vi "Process Script Check.vi"(8 "error in (no error)":errorcluster, 10 "Message":T1, 11 "Tamer in":refnum<class "Tamer.lvclass">=refnum) -> (0 "error out":errorcluster, 3 "Tamer out":refnum<class "Tamer.lvclass">)   [LabVIEW 2020, in "CIRCUS_uServices.lvlib" / "Holy Trinity.lvlib" / "Tamer.lvlib" / "Tamer.lvclass"]
uses:
  Tamer.lvclass
  TALOS/TALOS_PPL.lvlibp
  Run Utilities/TypeDefs/Script Checker Result.ctl
  Run Utilities/Run Utilities.lvlib
  Run Utilities/TypeDefs/Messages/Script Checker Message.ctl
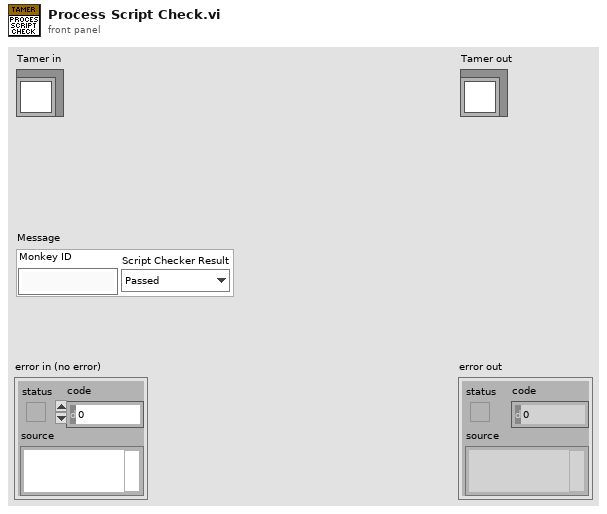
[diagram p1: front panel]
types:
  T1 = typedef "CIRCUS_uServices.lvlib/Run Utilities.lvlib/Script Checker Message.ctl" = cluster{"Monkey ID":string, "Script Checker Result":T2}
  T2 = typedef "CIRCUS_uServices.lvlib/Run Utilities.lvlib/Script Checker Result.ctl" = enum16{"Passed", "Failed", "Empty"}
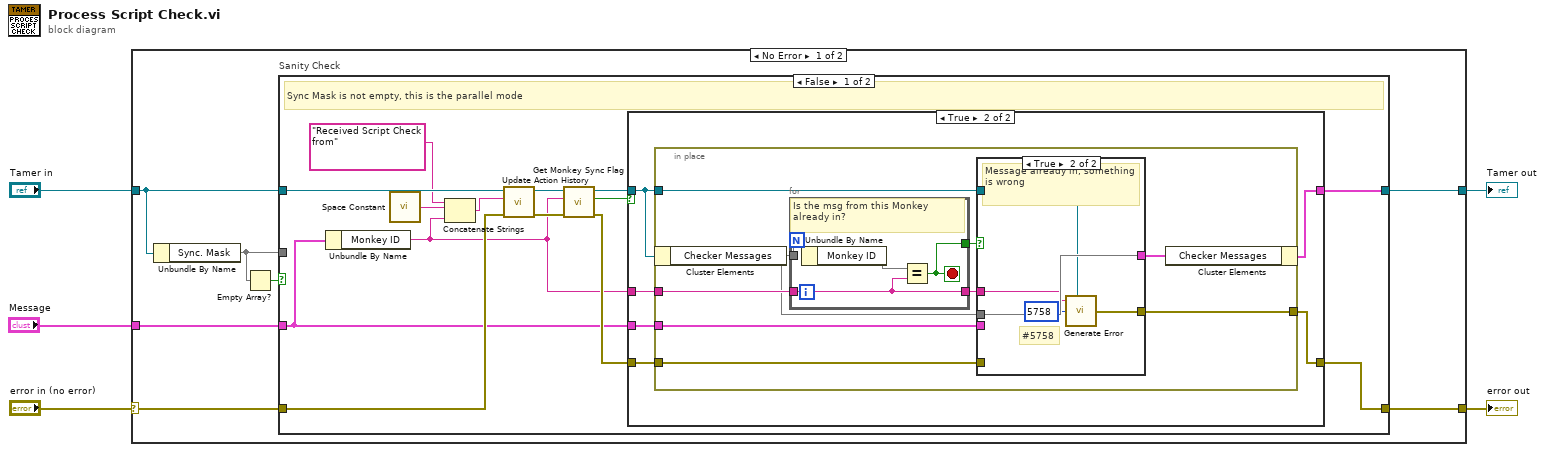
[diagram p0: block diagram]
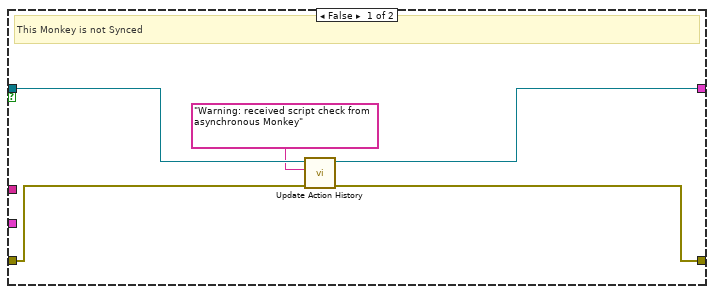
[diagram p2: hidden frame]
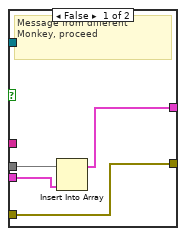
[diagram p3: hidden frame]
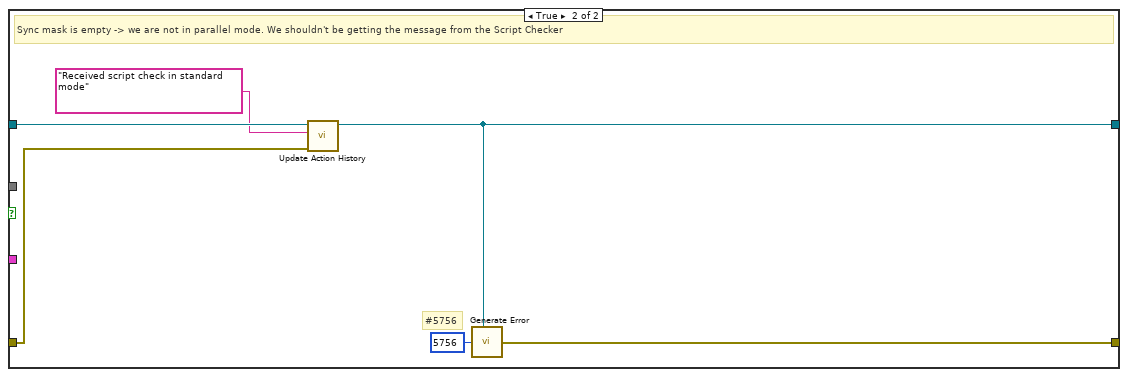
[diagram p4: hidden frame]
diagram:
  n1 = case shown="No Error" "error in (no error)" {
    selector: "error in (no error)" -> [w7 w67]
    tunnel: [w8 w67] -> w4
    tunnel: [w6 w66] -> w2
    tunnel: "Tamer in" -> [w9 w66]
    tunnel: "Message" -> [w12 _]
    frame No Error {
      n2 = Unbundle By Name(w9) -> ("Sync. Mask"=w10)
      n3 = Empty Array?(array=w10) -> (empty?=w11:bool)
      n4 = case "Sanity Check" shown="False" w11 {
        tunnel: w12 -> [w22 _]
        tunnel: w10 -> [_ _]
        tunnel: w9 -> [w18 w63]
        tunnel: [w21 w65] -> w8
        tunnel: w7 -> [w26 w60]
        tunnel: [w20 w62] -> w6
        frame False {
          # "Sync Mask is not empty, this is the parallel mode"
          n5 = Unbundle By Name(w22) -> ("Monkey ID"=w13:string)
          n6 = call <vilib>:"Space Constant.vi"() -> ("String"=w14:string)
          n7 = Concatenate Strings("Received Script Check from" ("string"), w14, w13) -> (w15:string)
          n8 = call-dynamic "Update Action History.vi"("error in (no error)"=w26, "Action"=w15, "Tamer in"=w18) -> ("error out"=w25:errorcluster, "Tamer out"=w17:refnum<class "Tamer.lvclass">)  [unwired: 7 in]
          n9 = call-dynamic "Get Monkey Sync Flag.vi"("error in (no error)"=w25, "Monkey ID"=w13, "Tamer in"=w17) -> ("error out"=w24:errorcluster, "Monkey Sync Flag"=w19:bool, "Tamer out"=w23:refnum<class "Tamer.lvclass">)  [unwired: 6 in]
          n10 = case shown="True" w19 {
            tunnel: w23 -> [w31 w35]
            tunnel: w22 -> [_ w37]
            tunnel: w13 -> [_ w36]
            tunnel: w24 -> [w29 w34]
            tunnel: [w28 w33] -> w21
            tunnel: [w30 w32] -> w20
            frame False {
              # "This Monkey is not Synced"
              n11 = call-dynamic "Update Action History.vi"("error in (no error)"=w29, "Action"="Warning: received script check from asynchronous Monkey", "Tamer in"=w31) -> ("error out"=w28:errorcluster, "Tamer out"=w30:refnum<class "Tamer.lvclass">)  [unwired: 7 in]
            }
            frame True {
              n12 = in-place {
                in-place-border: w37 -> [w44]
                in-place-border: w36 -> [w46]
                in-place-border: w35 -> [w41]
                in-place-border: w34 -> [w39]
                in-place-border: [w38] -> w33
                n13 = in-place-cluster #1(w35) -> ("Checker Messages"=w43)
                n14 = for {
                  tunnel: w43 -> [w59]
                  tunnel: w46 -> [w56]
                  tunnel: [w57] -> w45
                  tunnel: [w56] -> w40
                  stop <- w57 stop-if-true
                  # "Is the msg from this Monkey already in?"
                  n15 = Unbundle By Name(w59) -> ("Monkey ID"=w58)
                  n16 = Equal?(x=w58, y=w56) -> (x = y?=w57:bool)
                }
                n17 = case shown="True" w45 {
                  tunnel: w44 -> [w49 _]
                  tunnel: w43 -> [w50 w55]
                  tunnel: [w48 w55] -> w42
                  tunnel: w41 -> [_ w54]
                  tunnel: [w47 w53] -> w38
                  tunnel: w40 -> [_ w51]
                  tunnel: w39 -> [w47 _]
                  frame False {
                    # "Message from different Monkey, proceed"
                    n18 = Insert Into Array(array=w50, new element=w49) -> (w48:T1[])  [unwired: 1 in]
                  }
                  frame True {
                    # "#5758"
                    # "Message already in, something is wrong"
                    n19 = call "Generate Error.vi"("Optional String"=w51, "Class"=w54, "Error Code"=5758) -> ("error out"=w53:errorcluster)  [unwired: 4 in]
                  }
                }
                n20 = in-place-cluster #1("Checker Messages"=w42) -> (w32:cluster{})
              }
            }
          }
        }
        frame True {
          # "#5756"
          # "Sync mask is empty -> we are not in parallel mode. We shouldn't be getting the message from the Script Checker"
          n21 = call-dynamic "Update Action History.vi"("error in (no error)"=w60, "Action"="Received script check in standard mode", "Tamer in"=w63) -> ("Tamer out"=w62:refnum<class "Tamer.lvclass">)  [unwired: 7 in, 1 out]
          n22 = call "Generate Error.vi"("Class"=w62, "Error Code"=5756) -> ("error out"=w65:errorcluster)  [unwired: 5 in]
        }
      }
    }
    frame Error {
    }
  }
  "error out" <- w4
  "Tamer out" <- w2
